vi "Get SMO Public API.vi"(8 "error in (no error)":errorcluster, 11 "Instrument.Cryostat in":refnum<class "Instrument.Cryostat.lvclass">) -> (0 "error out":errorcluster, 2 "commands":string[](array[string]), 3 "Instrument.Cryostat out":refnum<class "Instrument.Cryostat.lvclass">)   [LabVIEW 2019, in "Instrument.Cryostat.lvclass"]
doc: "Override this VI to return a list of commands supported by your Instrument"
uses:
  Instrument.Cryostat.lvclass
  d7e12920-cb02-4624-bcd5-e5957f804813.vi
  Typedefs/Cryostat.commands--enum.ctl
  <userlib>/LevyLab/Instrument Framework/Instrument/Instrument.lvclass
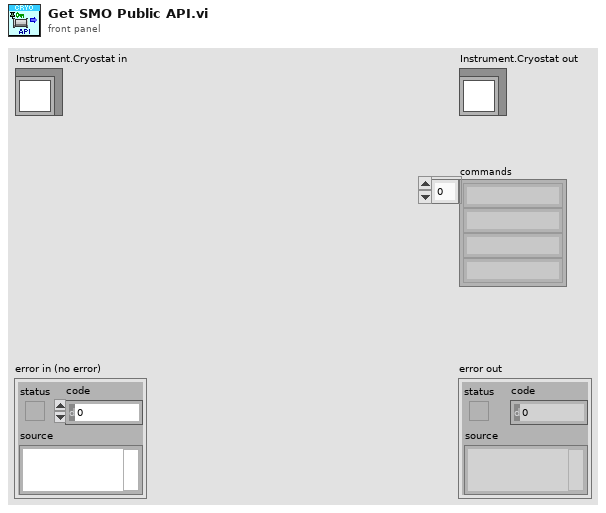
[diagram p1: front panel]
types:
  T1 = typedef "Instrument.Cryostat.lvclass/Cryostat.commands--enum.ctl" = enum16{"getLN2Level", "getLHeLevel", "getMagnet", "getMagnetVector", "setMagnet", "setMagnetVector", "getAngle", "setAngle", "getTemperature", "setTemperature", "getHeater", "setHeater", "getChamber", "setChamber", "getPressure"}
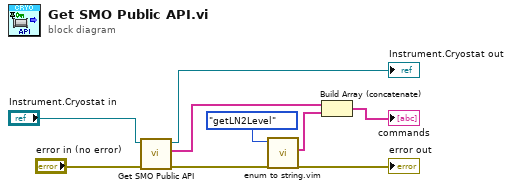
[diagram p0: block diagram]
diagram:
  n1 = call-parent "Get SMO Public API.vi"("error in (no error)"="error in (no error)", "Instrument in"="Instrument.Cryostat in") -> ("error out"=→"error out":errorcluster, "commands"=w2:string[], "Instrument out"=→"Instrument.Cryostat out":refnum<class "Instrument.Cryostat.lvclass">)  [unwired: 7 in]
  n2 = call "enum to string.vim"("enum in"=Cryostat.commands--enum."getLN2Level" ("commands")) -> ("strings out"=w4:string[])  [unwired: 9 in, 1 out]
  n3 = Build Array (concatenate)(w2, w4) -> (→"commands":string[])
